vi "Move Obj.vi"(7 "Direction":enum16{"Right", "Left", "Up", "Down"}(ring), 8 "error in (no error)":errorcluster, 10 "Magnitude":i32, 11 "Pane Object Position in":refnum<class "Pane Object Position.lvclass">) -> (0 "error out":errorcluster, 3 "Pane Object Position out":refnum<class "Pane Object Position.lvclass">)   [LabVIEW 2018, in "Pane Object Position.lvclass"]
uses:
  Pane Object Position.lvclass
  Pane Object Position.lvclass/Pane Object Position.ctl
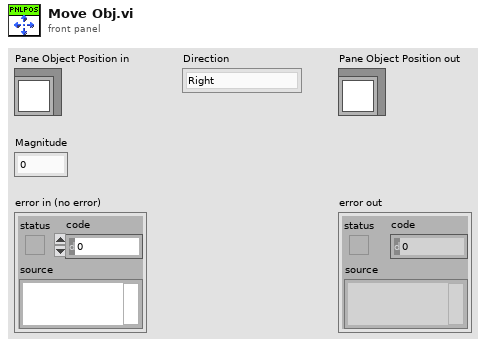
[diagram p1: front panel]
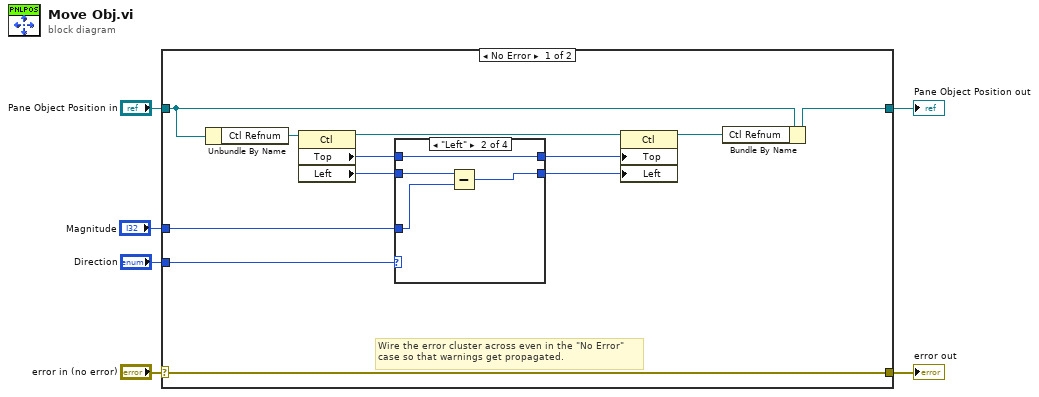
[diagram p0: block diagram]
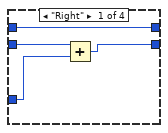
[diagram p2: hidden frame]
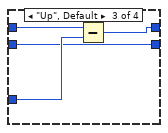
[diagram p3: hidden frame]
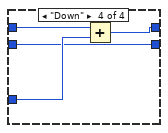
[diagram p4: hidden frame]
diagram:
  n1 = case shown="No Error" "error in (no error)" {
    selector: "error in (no error)" -> [w18 w36]
    tunnel: [w18 w36] -> w5
    tunnel: [w8 w35] -> w3
    tunnel: "Pane Object Position in" -> [w16 w35]
    tunnel: "Direction" -> [w13 _]
    tunnel: "Magnitude" -> [w12 _]
    frame No Error {
      # "Wire the error cluster across even in the \"No Error\"\ncase so that warnings get propagated."
      n2 = Unbundle By Name(w16) -> ("Ctl Refnum"=w17:refnum<vi>)
      n3 = property class="Ctl"(reference=w17) -> (reference out=w11:refnum<vi>, "Top"=w15:i32, "Left"=w14:i32)  [unwired: 1 in, 1 out]
      n4 = case shown="\"Left\"" w13 {
        tunnel: w15 -> [w19 w23 w30 w34]
        tunnel: w14 -> [w21 w26 w27 w31]
        tunnel: w12 -> [w22 w25 w29 w32]
        tunnel: [w20 w24 w27 w31] -> w9
        tunnel: [w19 w23 w28 w33] -> w10
        frame "Right" {
          n5 = Add(x=w21, y=w22) -> (x+y=w20:i32)
        }
        frame "Left" {
          n6 = Subtract(x=w26, y=w25) -> (x-y=w24:i32)
        }
        frame "Up", Default {
          n7 = Subtract(x=w30, y=w29) -> (x-y=w28:i32)
        }
        frame "Down" {
          n8 = Add(x=w34, y=w32) -> (x+y=w33:i32)
        }
      }
      n9 = property class="Ctl"(reference=w11, "Top"=w10, "Left"=w9) -> (reference out=w7:refnum<vi>)  [unwired: 1 in, 1 out]
      n10 = Bundle By Name(cluster=w16, "Ctl Refnum"=w7) -> (w8:refnum<class "Pane Object Position.lvclass">)
    }
    frame Error {
    }
  }
  "error out" <- w5
  "Pane Object Position out" <- w3
